vi "Close.vi"(8 "Error In":errorcluster, 11 "Xbox One Controller Ref":T1) -> (0 "Error Out":errorcluster)   [LabVIEW 2021, in "LMH-Xbox-One-Controller.lvlib"]
doc: "Close the connection to the Xbox controller."
uses:
  <instrlib>/Xbox-One-Controller/LMH-Xbox-One-Controller.lvlib
  <instrlib>/Xbox-One-Controller/Private/Type Defs/Xbox One Controller Ref.ctl
  <vilib>/Utility/inputDevices.llb/closeJoystick.vi
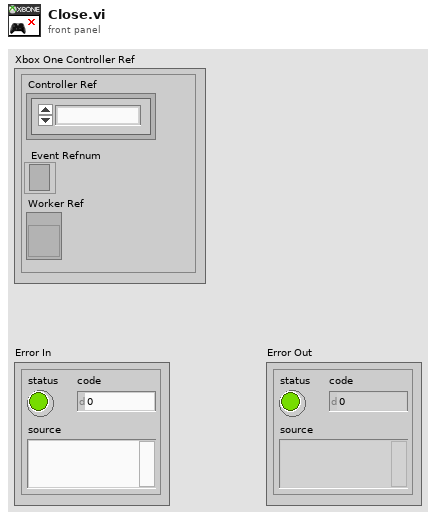
[diagram p1: front panel]
types:
  T1 = typedef "LMH-Xbox-One-Controller.lvlib/Xbox One Controller Ref.ctl" = cluster{"Controller Ref":refnum<k1>, "Event Refnum":refnum<event-registration>, "Worker Ref":refnum<vi>}
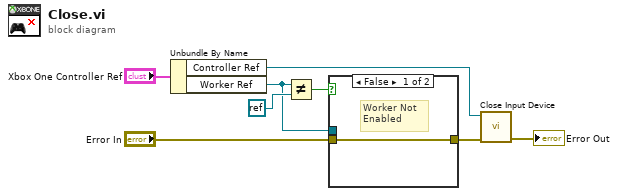
[diagram p0: block diagram]
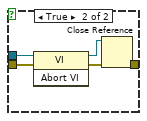
[diagram p2: hidden frame]
diagram:
  n1 = Unbundle By Name("Xbox One Controller Ref") -> ("Controller Ref"=w4:refnum<k1>, "Worker Ref"=w1:refnum<vi>)
  n2 = Not Equal?(x=w1, y=refnum<k0> refnum) -> (x != y?=w2:bool)
  n3 = case shown="False" w2 {
    tunnel: [w9 w12] -> w8
    tunnel: "Error In" -> [w9 w11]
    tunnel: w1 -> [_ w10]
    frame False {
      # "Worker Not \nEnabled"
    }
    frame True {
      n4 = invoke class="VI" method="Abort VI"(reference=w10, error in=w11) -> (reference out=w13:refnum<vi>, error out=w14:errorcluster)  [unwired: 1 in, 1 out]
      n5 = Close Reference(reference=w13, error in (no error)=w14) -> (error out=w12:errorcluster)
    }
  }
  n6 = call-poly <vilib>:"Close Input Device.vi"("error in (no error)"=w8, "device ID"=w4) -> ("error out"=→"Error Out":errorcluster)  [unwired: 8 in]
